vi "GetParam.vi"(8 "error in (no error)":errorcluster caption="entrée d'erreur (pas d'erreur)", 11 "power_transform.lvclass":refnum<class "power_transform.lvclass">) -> (0 "error out":errorcluster caption="sortie d'erreur", 2 "power_transform":T1={"method"="yeo-johnson", "standardize"=TRUE, "copy"=TRUE}, 3 "power_transform.lvclass":refnum<class "power_transform.lvclass">)   [LabVIEW 2020, in "power_transform.lvclass"]
doc: "Get Parameters"
uses:
  power_transform.lvclass
  power_transform.lvclass/power_transform.ctl
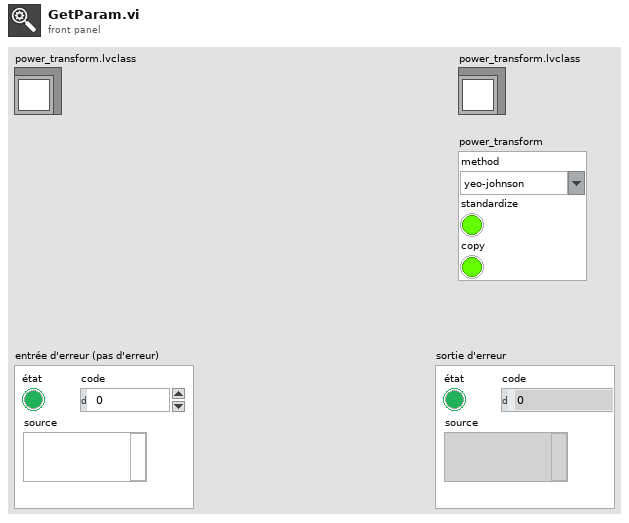
[diagram p1: front panel]
types:
  T1 = cluster{"method":string, "standardize":bool, "copy":bool}
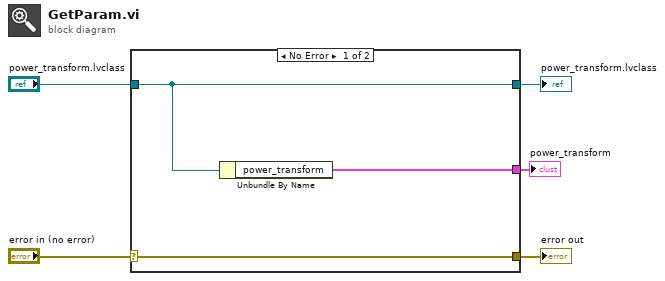
[diagram p0: block diagram]
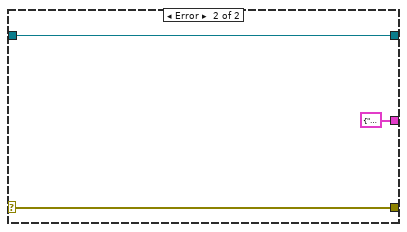
[diagram p2: hidden frame]
diagram:
  n1 = case shown="No Error" "error in (no error)" {
    selector: "error in (no error)" -> [w8 w10]
    tunnel: [w8 w10] -> w4
    tunnel: [w7 w11] -> w2
    tunnel: "power_transform.lvclass" -> [w7 w11]
    tunnel: [w6 T1 {"method"="", "standardize"=FALSE, "copy"=FALSE} ("power_transform")] -> w1
    frame No Error {
      n2 = Unbundle By Name(w7) -> ("power_transform"=w6:T1)
    }
    frame Error {
    }
  }
  "error out" <- w4
  "power_transform.lvclass" <- w2
  "power_transform" <- w1
